vi "Swerve Drive.vi"(11 "Drive Joystick":string="My Joystick RefNum") -> ()   [LabVIEW 2018]
uses:
  <vilib>/Rock Robotics/WPI/Utilities/WPI_GetSetVariantRefNum.vi
  <vilib>/Rock Robotics/Network Tables/NT Write Numeric Array.vi
  <vilib>/Rock Robotics/Network Tables/NT Write Number.vi
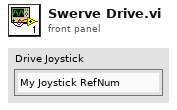
[diagram p1: front panel]
types:
  T1 = typedef "WPI_JoystickDevRef.ctl" = cluster{"Device":T2}
  T2 = typedef "WPI_JoystickDeviceEnum.ctl" = enum16{"USB 0", "USB 1", "USB 2", "USB 3", "USB 4", "USB 5"}
  T3 = cluster{"RL Angle":dbl, "RR Angle":dbl, "FL Angle":dbl, "FR Angle":dbl}
  T4 = cluster{"RR Drive Power":dbl, "FR Drive Power":dbl, "RL Drive Power":dbl, "FL Drive Power":dbl, "RL Steer Angle":dbl, "RR Steer Angle":dbl, "FL Steer Angle":dbl, "FR Steer Angle":dbl}
  T5 = cluster{"RR Drive Power":dbl, "FR Drive Power":dbl, "RL Drive Power":dbl, "FL Drive Power":dbl}
  T6 = cluster{"RR Error":dbl, "FR Error":dbl, "RL Error":dbl, "FL Error":dbl}
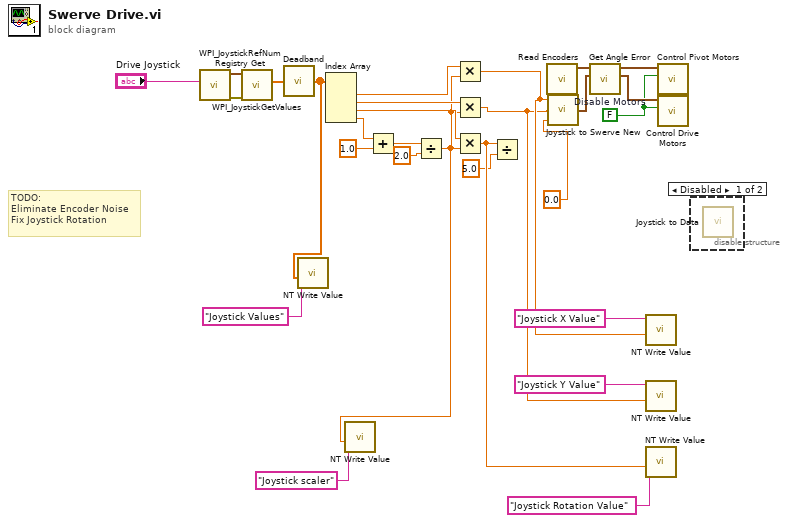
[diagram p0: block diagram]
diagram:
  w17 = FALSE  # Disable Motors
  # "TODO:\nEliminate Encoder Noise\nFix Joystick Rotation"
  n1 = call <vilib>:"WPI_JoystickRefNum Registry Get.vi"("refnum name"="Drive Joystick") -> ("error out"=w27:errorcluster, "JoystickDevRef"=w26:T1)  [unwired: 9 in]
  n2 = call <vilib>:"WPI_JoystickGetValues.vi"("error in (no error)"=w27, "JoystickDevRef"=w26) -> ("Axes"=w22:dbl[])  [unwired: 5 in, 4 out]
  n3 = call "Deadband.vi"("Axes"=w22) -> ("Deadbanded Axes"=w13:dbl[])
  n4 = call-poly <vilib>:"NT Write Value.vi"("Numeric Array"=w13, "Name"="Joystick Values") -> ()  [unwired: 9 in, 1 out]
  n5 = Index Array(array=w13) -> (element #1=w20:dbl, element #2=w19:dbl, element #3=w18:dbl, element #4=w16:dbl)  [unwired: 4 in]
  n6 = Add(x=w16, y=1.0) -> (x+y=w15:dbl)
  n7 = Divide(x=w15, y=2.0) -> (x/y=w8:dbl)
  n8 = call-poly <vilib>:"NT Write Value.vi"("Numeric"=w8, "Name"="Joystick scaler") -> ()  [unwired: 9 in, 1 out]
  n9 = Multiply(x=w20, y=w8) -> (x*y=w4:dbl)
  n10 = Multiply(x=w19, y=w8) -> (x*y=w3:dbl)
  n11 = Multiply(x=w18, y=w8) -> (x*y=w6:dbl)
  n12 = Divide(x=w6, y=5.0) -> ()  [unwired: 1 out]
  n13 = call "Read Encoders.vi"() -> ("Angles"=w25:T3)  [unwired: 11 in]
  n14 = call "Joystick to Swerve New.vi"("Joystick R"=0.0, "Joystick Y"=w3, "Joystick X"=w4) -> ("Swerve Data"=w1:T4)
  n15 = call "Get Angle Error.vi"("Goal Angles"=w1, "Real Angles"=w25) -> ("Motor Power"=w24:T5, "Angle Error"=w23:T6)  [unwired: 8 in]
  n16 = call-poly <vilib>:"NT Write Value.vi"("Numeric"=w4, "Name"="Joystick X Value") -> ()  [unwired: 9 in, 1 out]
  n17 = call-poly <vilib>:"NT Write Value.vi"("Numeric"=w3, "Name"="Joystick Y Value") -> ()  [unwired: 9 in, 1 out]
  n18 = call-poly <vilib>:"NT Write Value.vi"("Numeric"=w6, "Name"="Joystick Rotation Value") -> ()  [unwired: 9 in, 1 out]
  n19 = call "Control Pivot Motors.vi"("Disable Motors"=w17, "Cluster"=w23) -> ()  [unwired: 10 in]
  n20 = call "Control Drive Motors.vi"("Disable Motors"=w17, "Cluster"=w24) -> ()  [unwired: 10 in]
  n21 = disable-structure shown="Disabled" {
    frame Disabled {
      n22 = call "Joystick to Data.vi"() -> ()  [unwired: 3 in, 1 out]
    }
    frame Enabled {
    }
  }
